vi "CustomView.vi"(8 "error in":errorcluster, 10 "view name":string, 11 "CEF_Repository in":refnum<class "CEF_Repository.lvclass">) -> (0 "error out":errorcluster, 3 "CEF_Repository out":refnum<class "CEF_Repository.lvclass">)   [LabVIEW 2023, in "CEF.lvlib" / "CEF_Repository.lvclass"]
doc: "Calls the custom view specified in the view name string. The purpose of this method is to allow adding a Configurator editor without modifying the main VICopyright 2017 National Instruments Corporation\n\nLicensed under the Apache License, Version 2.0 (the \"License\"); you may not use this file except in compliance with the License. You may obtain a copy of the License at http://www.apache.org/licenses/LICENSE-2.0\nUnless required by applicable law or agreed to in writing, software distributed under the License is distributed on an \"AS IS\" BASIS, WITHOUT WARRANTIES OR CONDITIONS OF ANY KIND, either express or implied. See the License for the specific language governing permissions and limitations under the License."
uses:
  CEF_Repository.lvclass
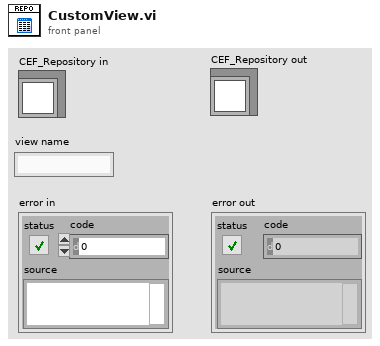
[diagram p1: front panel]
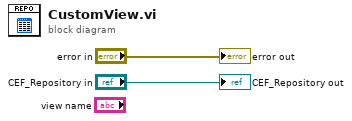
[diagram p0: block diagram]
diagram:
  "CEF_Repository out" <- "CEF_Repository in"
  "error out" <- "error in"
